vi "PR_Update_Error_Remove.vi"(7 "[workplace_id]":i16=5, 8 "error in (no error)":errorcluster, 9 "position":string="B", 10 "barcode":string="7890", 11 "DBlink":string="Driver={ODBC Driver 17 for SQL Server};Server=localhost\\SQLEXPRESS;Database=ZDX201;UID=labview;PWD=Dsa@54137926") -> (0 "error out":errorcluster)   [LabVIEW 2019]
uses:
  <vilib>/addons/database/Connection.llb/DB Tools Open Connec (String).vi
  <vilib>/addons/database/NI_Database_API.lvlib
panel:
  out "concatenated string":string="WHERE [barcode]='7890' and [position]='B'"
  in  "columns":string[](array[string])=["workspace_id", "time_spout"]
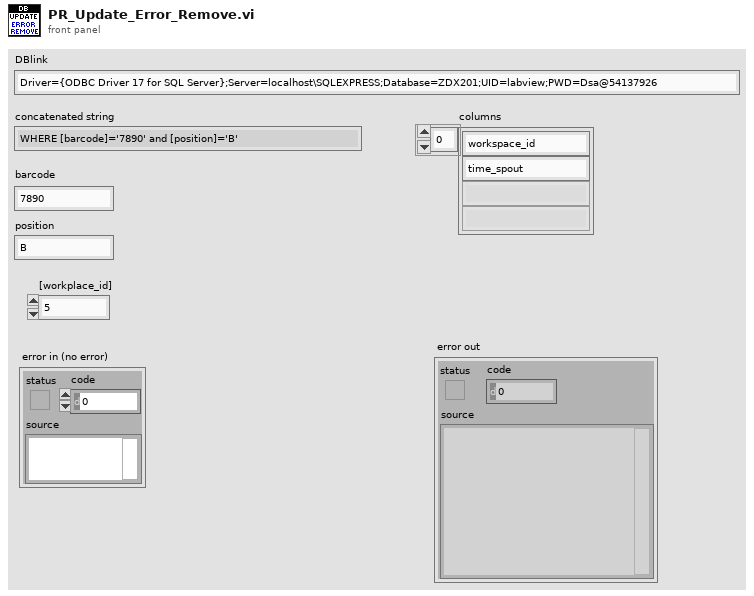
[diagram p1: front panel]
types:
  T1 = cluster{"[workplace_id]":i16, "spout_time":timestamp}
  T2 = typedef "NI_Database_API.lvlib/Conn ObjectReference.ctl" = refnum<k1>
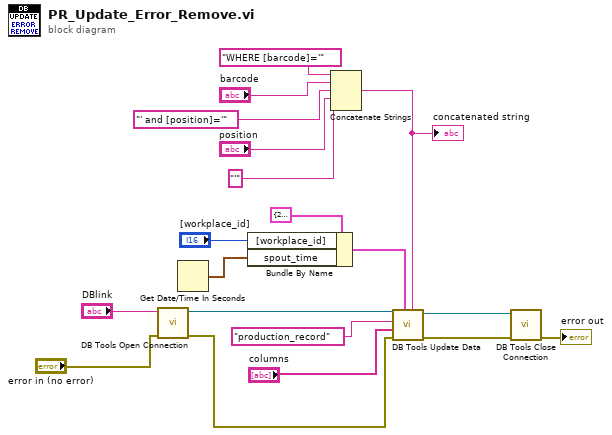
[diagram p0: block diagram]
diagram:
  n1 = call-poly <vilib>:"DB Tools Open Connection.vi"("error in (no error)"="error in (no error)", "connection information"="DBlink") -> ("error out"=w17:errorcluster, "connection reference"=w15:T2)  [unwired: 6 in]
  n2 = Get Date/Time In Seconds() -> (seconds since 1Jan1904=w2:timestamp)
  n3 = Bundle By Name(cluster=T1 {"[workplace_id]"=2, "spout_time"=timestamp(0 s since 1904-01-01)}, "[workplace_id]"="[workplace_id]", "spout_time"=w2) -> (w1:T1)
  n4 = Concatenate Strings("WHERE [barcode]='", "barcode", "' and [position]='" ("string"), "position", "'" ("string")) -> (w9:string)
  "concatenated string" <- w9
  n5 = call <vilib>:"DB Tools Update Data.vi"("condition"=w9, "data"=w1, "error in (no error)"=w17, "columns"="columns", "table"="production_record", "connection reference"=w15) -> ("error out"=w18:errorcluster, "connection reference out"=w16:T2)  [unwired: 4 in]
  n6 = call <vilib>:"DB Tools Close Connection.vi"("error in (no error)"=w18, "connection reference"=w16) -> ("error out"=→"error out":errorcluster)  [unwired: 5 in]
